vi "GetDigiRef.vi"(8 "error in (no error)":errorcluster, 11 "RIO Device IN":T2 caption="RIO Device") -> (0 "error out":errorcluster, 3 "FPGA VI Reference Out":T1)   [LabVIEW 2020]
uses:
  <vilib>/userdefined/High Color/nirio_resource_hc.ctl
  DigiFPGARef.ctl
  <vilib>/FPGAPlugInAG/PXIe-7962R/niLvFpga_Open_PXIe-7962R.vi
  <vilib>/rvi/interface/common/dynamic/niFpgaDynamicAddResources.vi
  <vilib>/rvi/interface/nirviOpenFPGA/nirviOpenFPGA.xnode
  FPGA Bitfiles/acoustoxv3_5772_Avg (Working).lvbitx
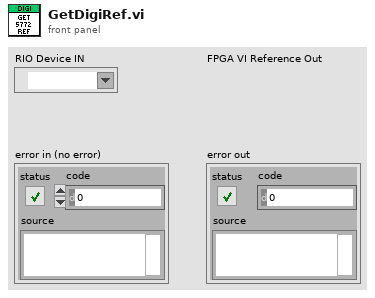
[diagram p1: front panel]
types:
  T1 = typedef "DigiFPGARef.ctl" = refnum<k20>
  T2 = typedef "nirio_resource_hc.ctl" = tag
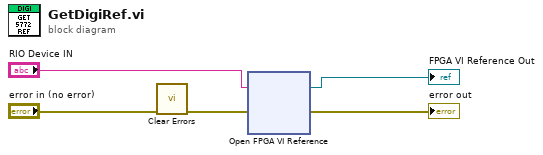
[diagram p0: block diagram]
diagram:
  n1 = call <vilib>:"Clear Errors.vi"("error in (no error)"="error in (no error)") -> ("error out"=w2:errorcluster)  [unwired: 5 in, 1 out]
  n2 = xnode "Open FPGA VI Reference"("error in"=w2, "resource name"="RIO Device IN") -> ("FPGA VI Reference Out"=→"FPGA VI Reference Out":refnum<k20>, "error out"=→"error out":errorcluster)
